vi "updateSpikeController.vi"(4 "Set Spike Position (in)":dbl(slide) scale=0.0..0.5, 6 "set Spike Position graph":dbl[](graph), 7 "distance to go":dbl caption="set Distance to Go (in)" format="%.3f", 8 "error in (no error)":errorcluster, 9 "set Motor Signal":string, 10 "set spike position":dbl format="%.3f", 11 "spikeController in":refnum<class "spikeController.lvclass">) -> (0 "error out":errorcluster, 3 "spikeController out":refnum<class "spikeController.lvclass">)   [LabVIEW 2025, in "spikeController.lvclass"]
uses:
  spikeController.lvclass
  spikeController.lvclass/spikeController.ctl
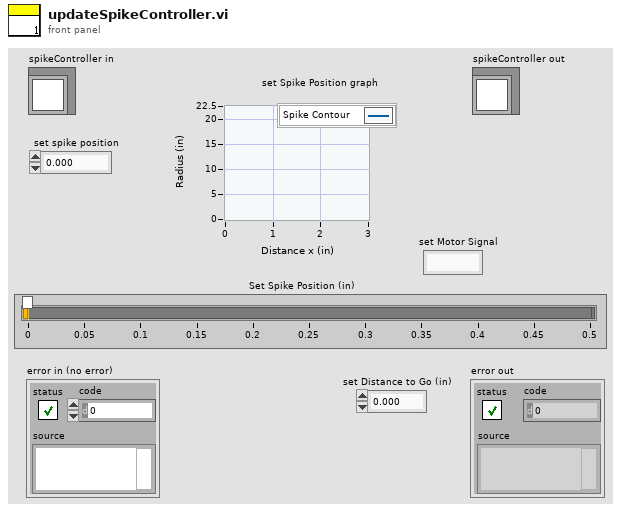
[diagram p1: front panel]
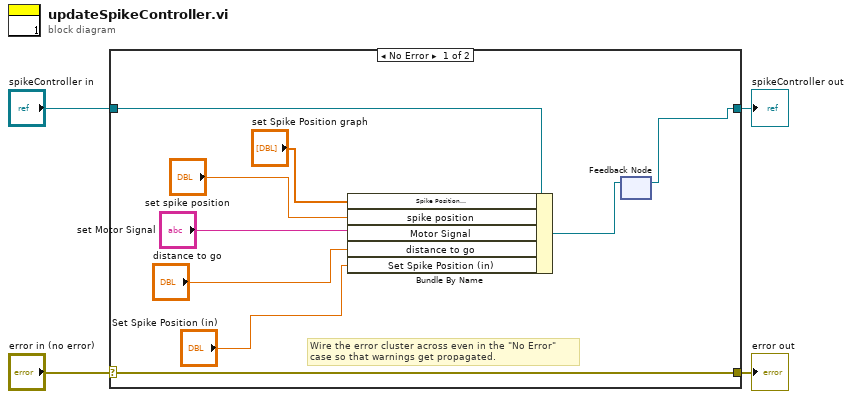
[diagram p0: block diagram]
diagram:
  n1 = case shown="No Error" "error in (no error)" {
    selector: "error in (no error)" -> [w13 w15]
    tunnel: [w13 w15] -> w3
    tunnel: [w11 w14] -> w1
    tunnel: "spikeController in" -> [w6 w14]
    frame No Error {
      # "Wire the error cluster across even in the \"No Error\"\ncase so that warnings get propagated."
      n2 = Bundle By Name(cluster=w6, "Spike Position \n(via Potentiometer)"="set Spike Position graph", "spike position"="set spike position", "Motor Signal"="set Motor Signal", "distance to go"="distance to go", "Set Spike Position (in)"="Set Spike Position (in)") -> (w12:refnum<class "spikeController.lvclass">)
      n3 = feedback-in #1(w12) -> ()
      n4 = feedback #1() -> (w11:refnum<class "spikeController.lvclass">)  [unwired: 1 in]
    }
    frame Error {
    }
  }
  "error out" <- w3
  "spikeController out" <- w1
